vi "ZMC Get Stop Pause Taskid.vi"(8 "error in (no error)":errorcluster caption="错误输入（无错误）", 10 "ptaskid":string, 11 "handle":u32) -> (0 "error out":errorcluster caption="错误输出", 1 "function return":i32, 2 "ptaskid out":string, 3 "handle out":u32)   [LabVIEW 2015, in "zauxdll.lvlib"]
doc: "int32 __stdcall ZMC_GetStopPauseTaskid(ZMC_HANDLE handle,uint8 *ptaskid);"
uses:
  zauxdll.lvlib
  zmotion.dll
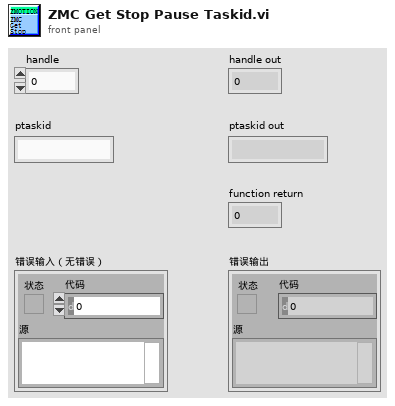
[diagram p1: front panel]
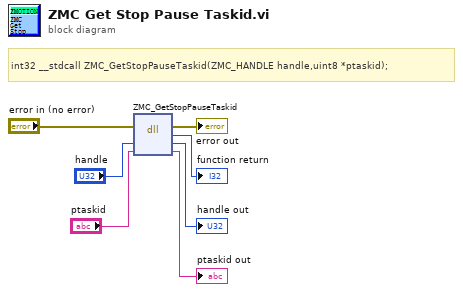
[diagram p0: block diagram]
diagram:
  # "int32 __stdcall ZMC_GetStopPauseTaskid(ZMC_HANDLE handle,uint8 *ptaskid);"
  n1 = dll-call lib="C:/Users/VIC/Desktop/GOGORO_SA/system/LLB/zmotion/zaux/zmotion.*" fn="ZMC_GetStopPauseTaskid"(error in="error in (no error)", "handle"="handle", "ptaskid"="ptaskid") -> (error out=→"error out":errorcluster, →"function return":i32, "handle"=→"handle out":u32, "ptaskid"=→"ptaskid out":string)  [unwired: 2 in, 1 out]
